vi "Read Location and Position Window.vi"(4 "Error In":errorcluster, 7 "VI Refnum":refnum<vi>) -> (0 "Error Out":errorcluster)   [LabVIEW 2014, in "User Interface.lvlib"]
uses:
  User Interface.lvlib
  <vilib>/Utility/sysdir.llb/System Directory Type.ctl
  <vilib>/Utility/config.llb/Read Key (String).vi
  <vilib>/Utility/config.llb/NI_LVConfig.lvlib
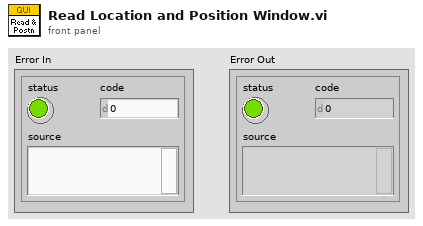
[diagram p1: front panel]
types:
  T1 = typedef "System Directory Type.ctl" = i32
  T2 = typedef "NI_LVConfig.lvlib/Config Data RefNum.ctl" = refnum<k1>
  T3 = typedef "LVRectTypeDef.ctl" = cluster{"Left":i16, "Top":i16, "Right":i16, "Bottom":i16}
  T4 = cluster{"Left":bool, "Top":bool, "Right":bool, "Bottom":bool}
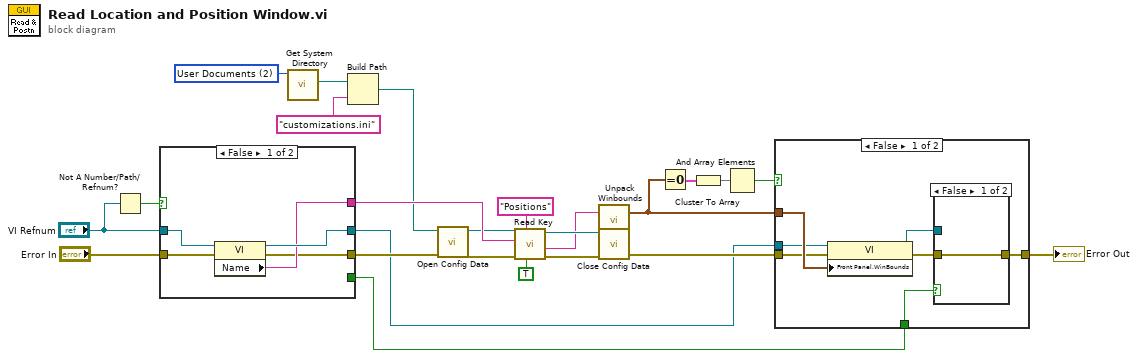
[diagram p0: block diagram]
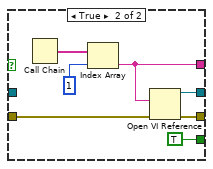
[diagram p2: hidden frame]
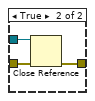
[diagram p3: hidden frame]
diagram:
  w4 = T1 2 items=["User Home"=0, "User Desktop"=1, "User Documents"=2, "User Application Data"=3, "User Preferences"=4, "User Temporary"=5, "Public Documents"=6, "Public Application Data"=7, "Public Preferences"=8, "Public Cache"=13, "System Core Libraries"=9, "System Installed Libraries"=10, "Application Files"=11, "Boot Volume Root"=12] ("system directory type")
  n1 = Not A Number/Path/Refnum?(number/path/refnum="VI Refnum") -> (NaN/Path/Refnum?=w19:bool)
  n2 = case shown="False" w19 {
    tunnel: [w26 w32] -> w22
    tunnel: "Error In" -> [w29 w34]
    tunnel: [w25 w33] -> w17
    tunnel: [w27 w31] -> w16
    tunnel: "VI Refnum" -> [w28 _]
    tunnel: [_ TRUE] -> w14
    frame False {
      n3 = property class="VI"(reference=w28, error in=w29) -> (reference out=w27:refnum<vi>, error out=w25:errorcluster, "Name"=w26:string)
    }
    frame True {
      n4 = Call Chain() -> (call chain=w36:string[])
      n5 = Index Array(array=w36, index=1) -> (element=w32:string)
      n6 = Open VI Reference(vi path=w32, error in (no error)=w34) -> (vi reference=w31:refnum<vi>, error out=w33:errorcluster)  [unwired: 4 in]
    }
  }
  n7 = call <vilib>:"Get System Directory.vi"("system directory type"=w4) -> ("system directory"=w3:path)  [unwired: 10 in]
  n8 = Build Path(base path=w3, name or relative path="customizations.ini") -> (appended path=w1:path)
  n9 = call <vilib>:"Open Config Data.vi"("error in (no error)"=w17, "configuration file path"=w1) -> ("error out"=w13:errorcluster, "refnum"=w12:T2)  [unwired: 7 in, 1 out]
  n10 = call-poly <vilib>:"Read Key.vi"("read raw string? (F)"=TRUE, "section"="Positions", "error in (no error)"=w13, "key"=w22, "refnum"=w12) -> ("error out"=w9:errorcluster, "value"=w7:string, "refnum out"=w8:T2)  [unwired: 3 in, 1 out]
  n11 = call "Unpack Winbounds.vi"("value"=w7) -> ("Front Panel.WinBounds"=w21:T3)  [unwired: 2 in]
  n12 = call <vilib>:"Close Config Data.vi"("error in (no error)"=w9, "refnum"=w8) -> ("error out"=w23:errorcluster)  [unwired: 8 in, 1 out]
  n13 = Equal To 0?(x=w21) -> (x = 0?=w6:T4)
  n14 = Cluster To Array(cluster=w6) -> (array=w5:bool[])
  n15 = And Array Elements(Boolean array=w5) -> (logical AND=w20:bool)
  n16 = case shown="False" w20 {
    tunnel: [w41 w48] -> w24
    tunnel: w23 -> [w38 w48]
    tunnel: w21 -> [w40 _]
    tunnel: w16 -> [w39 _]
    tunnel: w14 -> [w37 _]
    frame False {
      n17 = property class="VI"(reference=w39, error in=w38, "Front Panel.WinBounds"=w40) -> (reference out=w42:refnum<vi>, error out=w43:errorcluster)
      n18 = case shown="False" w37 {
        tunnel: w43 -> [w44 w47]
        tunnel: w42 -> [_ w46]
        tunnel: [w44 w45] -> w41
        frame False {
        }
        frame True {
          n19 = Close Reference(reference=w46, error in (no error)=w47) -> (error out=w45:errorcluster)
        }
      }
    }
    frame True {
    }
  }
  "Error Out" <- w24
